vi "AutoMatch.vi"() -> ()   [LabVIEW 2025]
panel:
  out "# of iterations":dbl
  in  "Number to Match":dbl
  out "Current Number":dbl
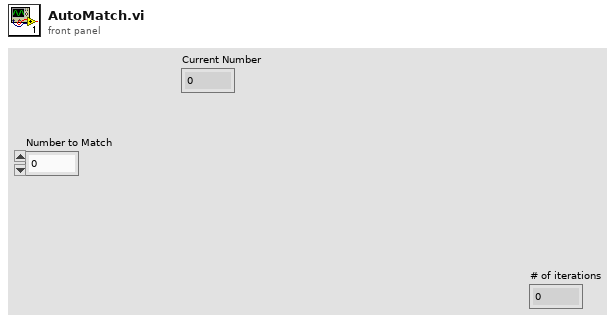
[diagram p1: front panel]
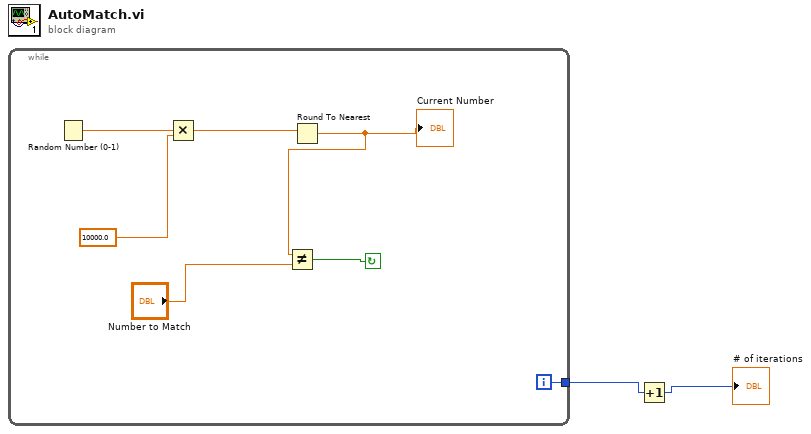
[diagram p0: block diagram]
diagram:
  n1 = while {
    tunnel: [w4] -> w2
    i -> [w4]
    stop <- w3 continue-if-true
    n2 = Random Number (0-1)() -> (number: 0 to 1=w9:dbl)
    n3 = Multiply(x=w9, y=10000.0) -> (x*y=w8:dbl)
    n4 = Round To Nearest(number=w8) -> (nearest integer value=w5:dbl)
    "Current Number" <- w5
    n5 = Not Equal?(x=w5, y="Number to Match") -> (x != y?=w3:bool)
  }
  n6 = Increment(x=w2) -> (x+1=→"# of iterations":i32)
